vi "U64 to U32.vi"(2 "error in (no error)":errorcluster, 3 "U64":dbl) -> (0 "error out":errorcluster, 1 "U32":u32)   [LabVIEW 2017]
panel:
  # "LVHDF5 Toolkit\nCopyright (c) 2005-2013 by Jason D. Sommerville\nCopyright (c) 2014 by UPVI, LLC.\n\nThis use and distribution of this file is governed by the terms found in \nLICENSE.txt distributed with this toolkit and installed at\n <user.lib>\\_lvhdf5\\LICENSE.txt"
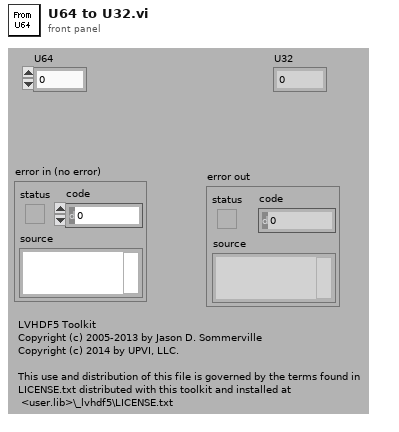
[diagram p1: front panel]
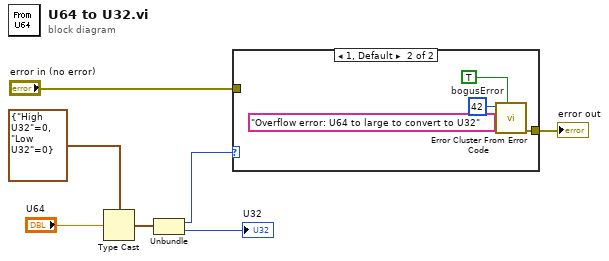
[diagram p0: block diagram]
diagram:
  n1 = Type Cast(type=cluster{"High U32":u32, "Low U32":u32} {"High U32"=0, "Low U32"=0}, x="U64") -> (*(type *) &x=w5:cluster{"High U32":u32, "Low U32":u32})
  n2 = Unbundle(w5) -> ("High U32"=w3:u32, "Low U32"=→"U32":u32)
  n3 = case shown="1, Default" w3 {
    tunnel: [w8 w9] -> w2
    tunnel: "error in (no error)" -> [w8 _]
    frame 0 {
    }
    frame 1, Default {
      w12 = 42  # bogusError
      n4 = call <vilib>:"Error Cluster From Error Code.vi"("show call chain? (False)"=TRUE, "error message (\"\")"="Overflow error: U64 to large to convert to U32" ("error message (\"\")"), "error code (0)"=w12) -> ("error out"=w9:errorcluster)  [unwired: 6 in]
    }
  }
  "error out" <- w2
